vi "GetTagValues_U8s.vi"(6 "error in (no error)":errorcluster caption="Fehler (Eingang, kein Fehler)", 7 "Tag Code":u16, 8 "Directory Entries":T2[](array[typedef]), 9 "TIFF file":T1 {"BigTiff,Endian" items=["Big-Endian"=0, "Native"=1, "Little-Endian"=2, "BigTiff-Big-Endian"=256, "Bigtiff,Native"=257, "Biftiff,Littleendian"=258]}) -> (0 "error out":errorcluster caption="Fehler (Ausgang)", 1 "Index (not found = -1)":i32, 2 "Byte array":u8[](array[numeric]), 3 "TIFF file out":T1 {"BigTiff,Endian" items=["Big-Endian"=0, "Native"=1, "Little-Endian"=2, "BigTiff-Big-Endian"=256, "Bigtiff,Native"=257, "Biftiff,Littleendian"=258]})   [LabVIEW 2011]
uses:
  IFD.ctl
panel:
  # "Oh dear if count >1 it may be an offset! (more than 32 bit)"
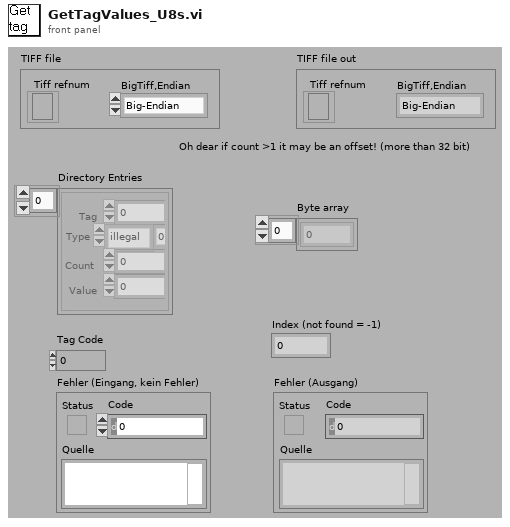
[diagram p1: front panel]
types:
  T1 = cluster{"Tiff refnum":refnum<file>, "BigTiff,Endian":u16}
  T2 = typedef "IFD.ctl" = cluster{"Tag":u16, "Type":enum16{"illegal", "Byte", "Ascii", "Short", "Long", "Rational", "SByte", "Undefined", "SShort", "SLong", "SRational 2xSLong", "Float 4byte", "Double 8Byte", "No13", "No14", "No15", "U64", "I64", "U64-IFD8"}, "Count":u64, "Value":u64}
  T3 = enum16{"illegal", "Byte", "Ascii", "Short", "Long", "Rational", "SByte", "Undefined", "SShort", "SLong", "SRational 2xSLong", "Float 4byte", "Double 8Byte"}[]
  T4 = enum16{"illegal", "Byte", "Ascii", "Short", "Long", "Rational", "SByte", "Undefined", "SShort", "SLong", "SRational 2xSLong", "Float 4byte", "Double 8Byte", "No13", "No14", "No15", "U64", "I64", "U64-IFD8"}
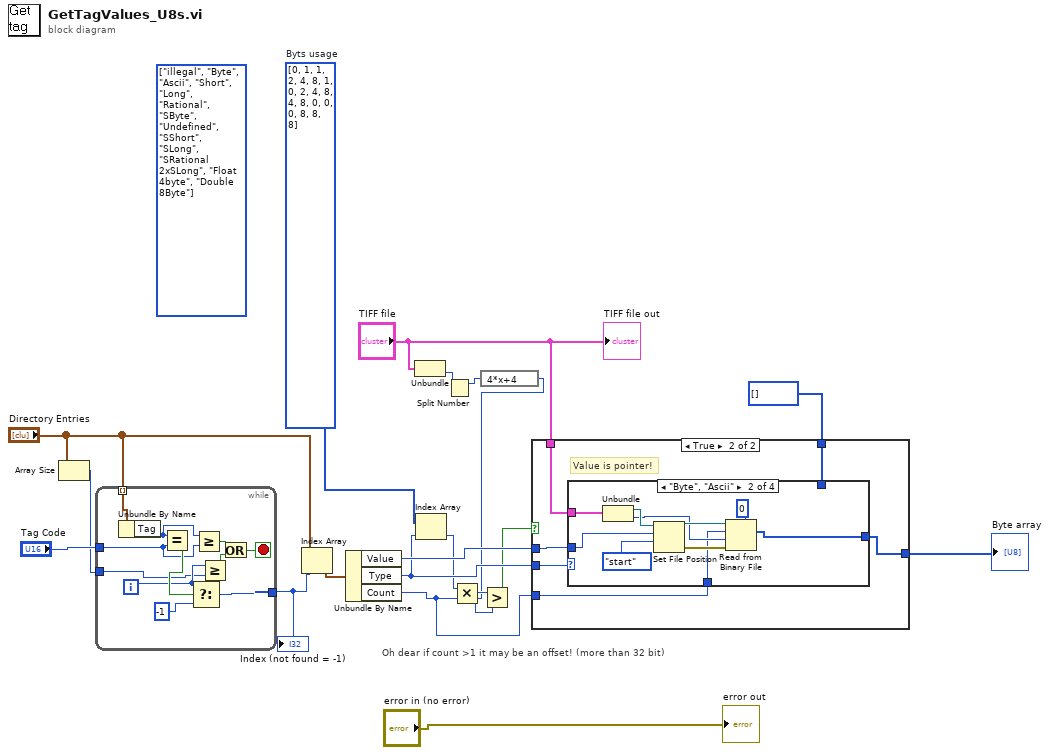
[diagram p0: block diagram]
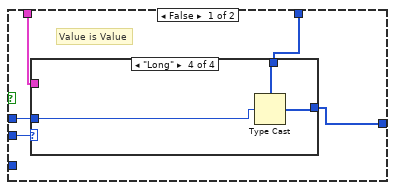
[diagram p2: hidden frame]
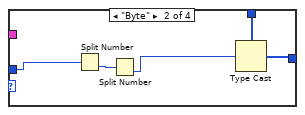
[diagram p4: hidden frame]
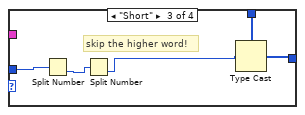
[diagram p5: hidden frame]
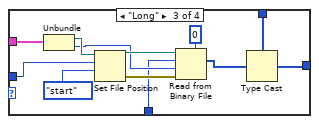
[diagram p7: hidden frame]
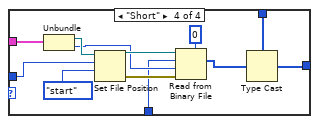
[diagram p8: hidden frame]
diagram:
  w6 = i32[] [0, 1, 1, 2, 4, 8, 1, 0, 2, 4, 8, 4, 8, 0, 0, 0, 8, 8, 8]  # Byts usage
  (unwired) T3 [enum."illegal", enum."Byte", enum."Ascii", enum."Short", enum."Long", enum."Rational", enum."SByte", enum."Undefined", enum."SShort", enum."SLong", enum."SRational 2xSLong", enum."Float 4byte", enum."Double 8Byte"] items=["illegal", "Byte", "Ascii", "Short", "Long", "Rational", "SByte", "Undefined", "SShort", "SLong", "SRational 2xSLong", "Float 4byte", "Double 8Byte"]
  # "Oh dear if count >1 it may be an offset! (more than 32 bit)"
  n1 = Array Size(array="Directory Entries") -> (size(s)=w14:i32)
  n2 = while {
    tunnel: "Directory Entries" -> [w30] mode=indexing
    tunnel: "Tag Code" -> [w27]
    tunnel: [w25] -> w16
    tunnel: w14 -> [w23]
    i -> [w24]
    stop <- w22 stop-if-true
    n3 = Unbundle By Name(w30) -> ("Tag"=w28:u16)
    n4 = Equal?(x=w28, y=w27) -> (x = y?=w29:bool)
    n5 = Select(t=w24, s=w29, f=-1) -> (s? t:f=w25:i32)
    n6 = Greater Or Equal?(x=w28, y=w27) -> (x >= y?=w21:bool)
    n7 = Greater Or Equal?(x=w24, y=w23) -> (x >= y?=w20:bool)
    n8 = Or(x=w21, y=w20) -> (x .or. y?=w22:bool)
  }
  "Index (not found = -1)" <- w16
  n9 = Index Array(array="Directory Entries", index=w16) -> (element=w18:T2)
  n10 = Unbundle By Name(w18) -> ("Value"=w17:u64, "Type"=w13:T4, "Count"=w9:u64)
  n11 = Unbundle("TIFF file") -> ("BigTiff,Endian"=w5:u16)  [unwired: 1 out]
  n12 = Index Array(array=w6, index=w13) -> (element=w12:i32)
  n13 = Split Number(x=w5) -> (hi(x)=w4:u8)  [unwired: 1 out]
  n14 = Multiply(x=w12, y=w9) -> (x*y=w11:u64)
  n15 = expression code="4*x+4"(w4) -> (w2:u8)
  n16 = Greater?(x=w11, y=w2) -> (0:w10:bool)
  n17 = case shown="True" w10 {
    tunnel: w17 -> [w35 w54]
    tunnel: "TIFF file" -> [w34 w55]
    tunnel: w13 -> [w33 w53]
    tunnel: [w32 w52] -> w8
    tunnel: w9 -> [_ w51]
    tunnel: u8[] [] -> [w31 w50]
    frame False {
      # "Value is Value"
      n18 = case shown="\"Long\"" w33 {
        tunnel: w34 -> [_ _ _ _]
        tunnel: w35 -> [_ w41 w43 w47]
        tunnel: [w36 w40 w45 w48] -> w32
        tunnel: w31 -> [w36 w39 w44 w49]
        frame "illegal", Default {
        }
        frame "Byte" {
          n19 = Split Number(x=w41) -> (lo(x)=w38:u32)  [unwired: 1 out]
          n20 = Split Number(x=w38) -> (lo(x)=w37:u16)  [unwired: 1 out]
          n21 = Type Cast(type=w39, x=w37) -> (*(type *) &x=w40:u8[])
        }
        frame "Short" {
          # "skip the higher word!"
          n22 = Split Number(x=w43) -> (lo(x)=w42:u32)  [unwired: 1 out]
          n23 = Split Number(x=w42) -> (lo(x)=w46:u16)  [unwired: 1 out]
          n24 = Type Cast(type=w44, x=w46) -> (*(type *) &x=w45:u8[])
        }
        frame "Long" {
          n25 = Type Cast(type=w49, x=w47) -> (*(type *) &x=w48:u8[])
        }
      }
    }
    frame True {
      # "Value is pointer!"
      n26 = case shown="\"Byte\", \"Ascii\"" w53 {
        tunnel: w55 -> [_ w60 w73 w85]
        tunnel: w54 -> [_ w59 w72 w84]
        tunnel: [w56 w58 w68 w80] -> w52
        tunnel: w51 -> [_ w57 w70 w82]
        tunnel: w50 -> [w56 _ w67 w79]
        frame "illegal", Default {
        }
        frame "Byte", "Ascii" {
          n27 = Unbundle(w60) -> ("Tiff refnum"=w63:refnum<file>, "BigTiff,Endian"=w62:u16)
          n28 = Set File Position(offset (in bytes) (0)=w59, refnum=w63, from (0:start)=enum16{"start", "end", "current"}."start" ("pos mode (0:2)")) -> (refnum out=w65:refnum<file>, error out=w64:errorcluster)  [unwired: 1 in]
          n29 = Read from Binary File(5:u8 0 ("byte stream type"), 8:w64, 9:w62, 10:w57, 11:w65) -> (2:w58:u8[])  [unwired: 4 out]
        }
        frame "Long" {
          n30 = Unbundle(w73) -> ("Tiff refnum"=w75:refnum<file>, "BigTiff,Endian"=w74:u16)
          n31 = Set File Position(offset (in bytes) (0)=w72, refnum=w75, from (0:start)=enum16{"start", "end", "current"}."start" ("pos mode (0:2)")) -> (refnum out=w77:refnum<file>, error out=w76:errorcluster)  [unwired: 1 in]
          n32 = Read from Binary File(5:u32 0 ("byte stream type"), 8:w76, 9:w74, 10:w70, 11:w77) -> (2:w69:u32[])  [unwired: 4 out]
          n33 = Type Cast(type=w67, x=w69) -> (*(type *) &x=w68:u8[])
        }
        frame "Short" {
          n34 = Unbundle(w85) -> ("Tiff refnum"=w87:refnum<file>, "BigTiff,Endian"=w86:u16)
          n35 = Set File Position(offset (in bytes) (0)=w84, refnum=w87, from (0:start)=enum16{"start", "end", "current"}."start" ("pos mode (0:2)")) -> (refnum out=w89:refnum<file>, error out=w88:errorcluster)  [unwired: 1 in]
          n36 = Read from Binary File(5:u16 0 ("byte stream type"), 8:w88, 9:w86, 10:w82, 11:w89) -> (2:w81:u16[])  [unwired: 4 out]
          n37 = Type Cast(type=w79, x=w81) -> (*(type *) &x=w80:u8[])
        }
      }
    }
  }
  "Byte array" <- w8
  "error out" <- "error in (no error)"
  "TIFF file out" <- "TIFF file"
